vi "Write Sequence index.vi"(8 "error in (no error)":errorcluster, 10 "Sequence index":i32=-1, 11 "PD-Data in":refnum<class "PD-Main.lvclass">) -> (0 "error out":errorcluster, 3 "PD-Data out":refnum<class "PD-Main.lvclass">)   [LabVIEW 2013, in "PowderDeposition.lvlib" / "PD-Main.lvclass"]
uses:
  PD-Main.lvclass
  PD-Main.lvclass/PD-Main.ctl
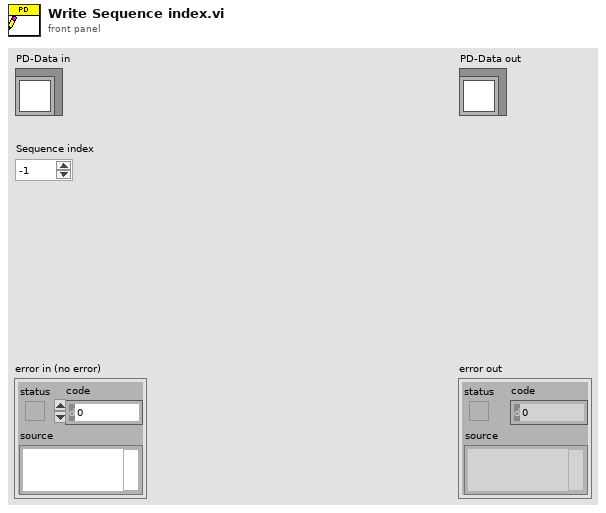
[diagram p1: front panel]
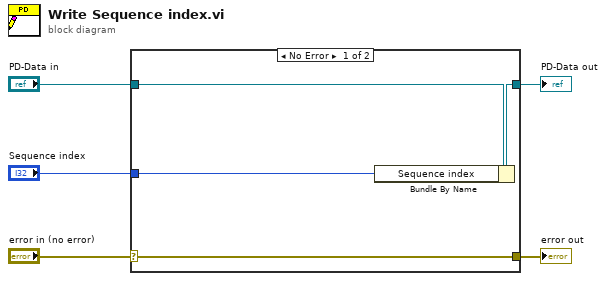
[diagram p0: block diagram]
diagram:
  n1 = case shown="No Error" "error in (no error)" {
    selector: "error in (no error)" -> [w9 w10]
    tunnel: [w9 w10] -> w4
    tunnel: [w7 w11] -> w2
    tunnel: "PD-Data in" -> [w8 w11]
    tunnel: "Sequence index" -> [w6 _]
    frame No Error {
      n2 = Bundle By Name(cluster=w8, "Sequence index"=w6) -> (w7:refnum<class "PD-Main.lvclass">)
    }
    frame Error {
    }
  }
  "error out" <- w4
  "PD-Data out" <- w2
